vi "Configure Offset Calculate Block.vi"(7 "Enable Offset (F: Disable)":bool, 8 "error in (no error)":errorcluster, 9 "Block Offset (0 dB)":dbl, 10 "Calculate Block (1: Calculate Block 1)":i32(ring)=1 items=["Calculate Block 1"=1, "Calculate Block 2"=2, "Calculate Block 3"=3, "Calculate Block 4"=4], 11 "VISA resource name":refnum<visa-resource-name>) -> (0 "error out":errorcluster, 3 "VISA resource name out":refnum<visa-resource-name>)   [LabVIEW 2018, in "Agilent U2000 Series.lvlib"]
doc: "Configures the offset on the specified calculate block. The offset is applied to the measurement signal after any math calculation."
uses:
  Agilent U2000 Series.lvlib
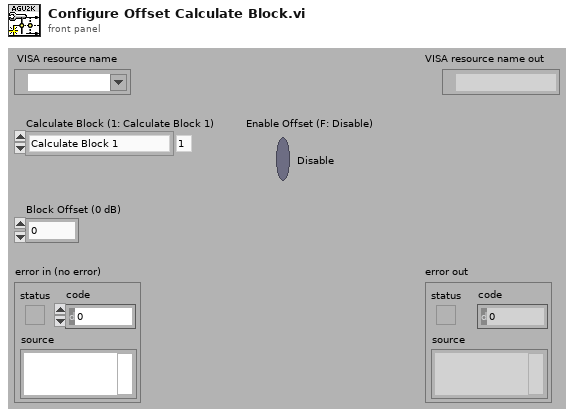
[diagram p1: front panel]
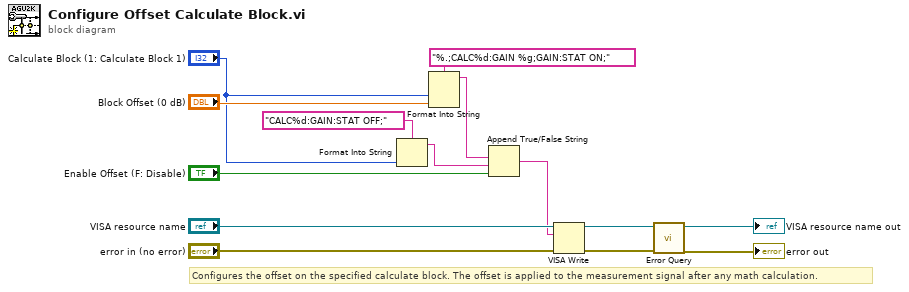
[diagram p0: block diagram]
diagram:
  # "Configures the offset on the specified calculate block. The offset is applied to the measurement signal after any math calculation."
  n1 = Format Into String(format string="CALC%d:GAIN:STAT OFF;", "Calculate Block (1: Calculate Block 1)") -> (resulting string=w2:string)  [unwired: 2 in, 1 out]
  n2 = Format Into String(format string="%.;CALC%d:GAIN %g;GAIN:STAT ON;", "Calculate Block (1: Calculate Block 1)", "Block Offset (0 dB)") -> (resulting string=w1:string)  [unwired: 2 in, 1 out]
  n3 = Append True/False String(1:"Enable Offset (F: Disable)", 2:w2, 3:w1) -> (0:w6:string)  [unwired: 1 out]
  n4 = VISA Write(VISA resource name="VISA resource name", write buffer=w6, error in (no error)="error in (no error)") -> (VISA resource name out=w10:refnum<visa-resource-name>, error out=w9:errorcluster)  [unwired: 1 out]
  n5 = call "Error Query.vi"("error in (no error)"=w9, "VISA resource name"=w10) -> ("error out"=→"error out":errorcluster, "VISA resource name out"=→"VISA resource name out":refnum<visa-resource-name>)  [unwired: 8 out]
